vi "StartDataCollectionWithTrigger.vi"(8 "error in (no error)":errorcluster, 10 "Points":i32=1000, 11 "controller in":refnum<k24>) -> (0 "error out":errorcluster, 3 "controller out":refnum<k24>)   [LabVIEW 2010]
uses:
  c:/aerotech/controller/dev/A3200/pc/labview/2010/bin/Aerotech.A3200.dll
  bin/Aerotech.A3200.dll
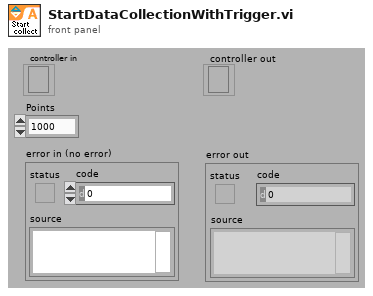
[diagram p1: front panel]
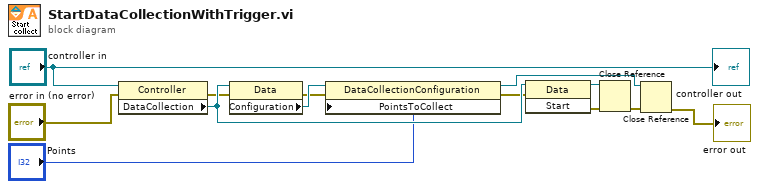
[diagram p0: block diagram]
diagram:
  n1 = property class="Controller"(reference="controller in", error in="error in (no error)") -> (error out=w7:errorcluster, "DataCollection"=w9:refnum<k24>)  [unwired: 1 out]
  n2 = property class="Data"(reference=w9, error in=w7) -> (error out=w1:errorcluster, "Configuration"=w2:refnum<k24>)  [unwired: 1 out]
  n3 = property class="DataCollectionConfiguration"(reference=w2, error in=w1, "PointsToCollect"="Points") -> (reference out=w4:refnum<k24>, error out=w5:errorcluster)
  n4 = invoke class="Data" method="Start"(reference=w9, error in=w5) -> (reference out=w10:refnum<k24>, error out=w11:errorcluster)  [unwired: 1 in, 1 out]
  n5 = Close Reference(reference=w10, error in (no error)=w11) -> (error out=w6:errorcluster)
  n6 = Close Reference(reference=w4, error in (no error)=w6) -> (error out=→"error out":errorcluster)
  "controller out" <- "controller in"
